vi "test.vi"() -> ()   [LabVIEW 2014]
uses:
  Array-Parameter/_support/Def-MassDataOper-Status.ctl
  Array-Parameter/_support/Operation-FGV-MassData.ctl
  Array-Parameter/JKISM++ Array Parameter Support.lvlib
panel:
  out "Waveform Graph":dbl[](graph)
  in  "Start":i32
  in  "read":bool
  out "Thermometer":cluster{dbl, dbl, dbl, dbl}(slide)={0.0, 6224.489795918367, 0.0, 0.0} scale=0.0..10000000.0
  in  "write":bool
  out "Active Read Oper":T1
  out "Active Write Oper":T1
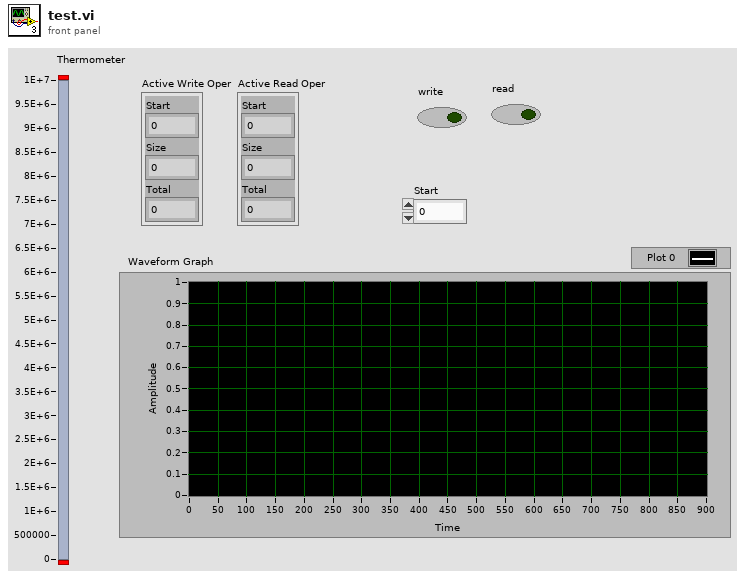
[diagram p1: front panel]
types:
  T1 = typedef "JKISM++ Array Parameter Support.lvlib/Def-MassDataOper-Status.ctl" = cluster{"Start":i32, "Size":i32, "Total":i32}
  T2 = typedef "JKISM++ Array Parameter Support.lvlib/Operation-FGV-MassData.ctl" = enum16{"Initialize", "Read", "Write", "Status", "Release"}
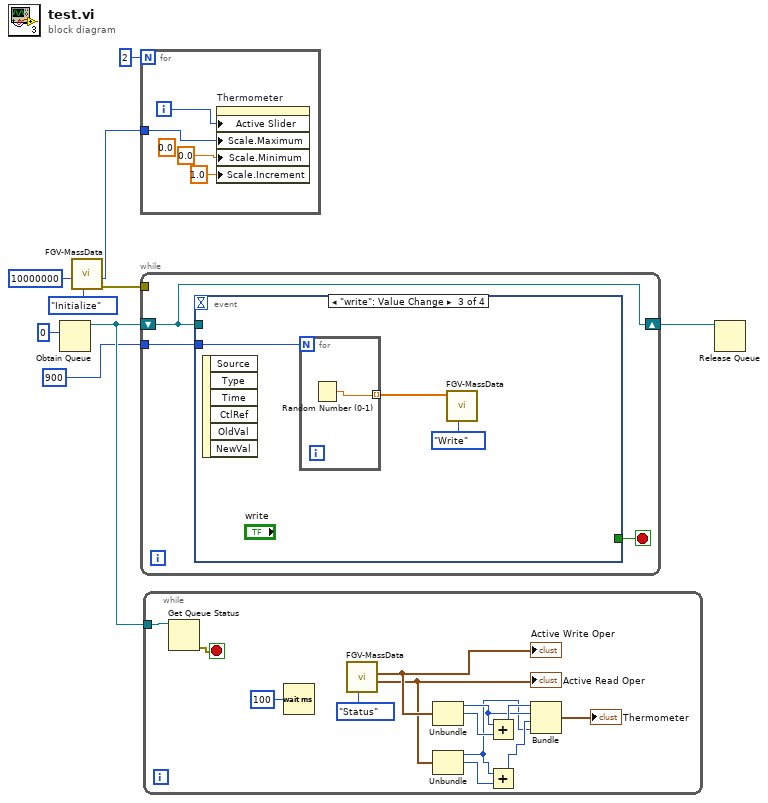
[diagram p0: block diagram]
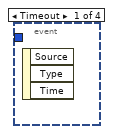
[diagram p2: hidden frame]
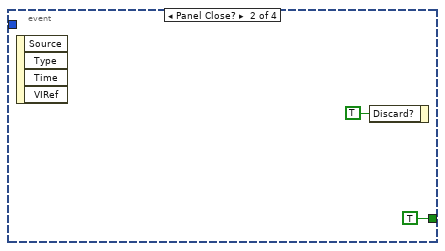
[diagram p3: hidden frame]
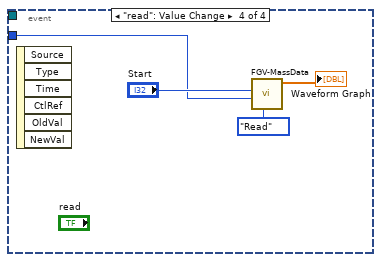
[diagram p4: hidden frame]
diagram:
  w2 = 10000000 ("size")
  n1 = Obtain Queue(element data type=0 ("size")) -> (queue out=w5:refnum<queue>)  [unwired: 4 in, 2 out]
  n2 = call "FGV-MassData.vi"("Operation"=Operation-FGV-MassData."Initialize", "size"=w2) -> ("Error out"=w7:errorcluster)  [unwired: 6 in, 3 out]
  n3 = for {
    N: 2 -> [_]
    tunnel: w2 -> [w10]
    i -> [w9]
    (unwired) 0.0 ("Scale.Range:Minimum")
    n4 = property on="Thermometer" class="Slide (strict)"("Active Slider"=w9, "Scale.Maximum"=w10, "Scale.Minimum"=0.0 ("Scale.Range:Minimum"), "Scale.Increment"=1.0 ("Scale.Range:Increment")) -> ()  [unwired: 2 in, 2 out]
  }
  n5 = while {
    tunnel: w7 -> [_]
    shift-right: [w14] -> w6
    shift-left: w5 -> [w14]
    tunnel: 900 -> [w13]
    stop <- w15 stop-if-true
    n6 = event shown="[2] \"write\": Value Change" {
      selector: _ -> [_ _ _ _]
      dyn-events: _ -> [_ _ _ _]
      timeout: _ -> [_ _ _ _]
      tunnel: [_ TRUE ("Discard?") _ _] -> w15
      tunnel: w14 -> [_ _ _ _]
      tunnel: w13 -> [_ _ w18 w23]
      event Timeout {
        n7 = event-data() -> ()  [unwired: 1 in, 3 out]
      }
      event Panel Close? {
        n8 = event-data() -> ()  [unwired: 1 in, 4 out]
        n9 = event-data("Discard?"=TRUE) -> ()  [unwired: 1 in, 1 out]
      }
      event "write": Value Change {
        n10 = event-data() -> ()  [unwired: 1 in, 6 out]
        n11 = for {
          N: w18 -> [_]
          tunnel: [w21] -> w19 mode=indexing
          n12 = Random Number (0-1)() -> (number: 0 to 1=w21:dbl)
        }
        n13 = call "FGV-MassData.vi"("Operation"=Operation-FGV-MassData."Write", "Data in"=w19) -> ()  [unwired: 6 in, 4 out]
      }
      event "read": Value Change {
        n14 = event-data() -> ()  [unwired: 1 in, 6 out]
        n15 = call "FGV-MassData.vi"("Operation"=Operation-FGV-MassData."Read", "size"=w23, "Start"="Start") -> ("Data out"=→"Waveform Graph":dbl[])  [unwired: 5 in, 3 out]
      }
    }
  }
  n16 = while {
    tunnel: w5 -> [w38]
    stop <- w37 stop-if-true
    n17 = Get Queue Status(queue=w38) -> (error out=w37:errorcluster)  [unwired: 2 in, 7 out]
    n18 = Wait (ms)(milliseconds to wait=u32 100) -> ()  [unwired: 1 out]
    n19 = call "FGV-MassData.vi"("Operation"=Operation-FGV-MassData."Status") -> ("Active Read Oper"=w29:T1, "Active Write Oper"=w34:T1)  [unwired: 7 in, 2 out]
    "Active Write Oper" <- w34
    "Active Read Oper" <- w29
    n20 = Unbundle(w34) -> ("Start"=w31:i32, "Size"=w33:i32)  [unwired: 1 out]
    n21 = Unbundle(w29) -> ("Start"=w27:i32, "Size"=w30:i32)  [unwired: 1 out]
    n22 = Add(x=w31, y=w33) -> (x+y=w32:i32)
    n23 = Add(x=w27, y=w30) -> (x+y=w28:i32)
    n24 = Bundle(w32, "Start"=w31, w28, "Start"=w27) -> (→"Thermometer":cluster{i32, "Start":i32, i32, "Start":i32})  [unwired: 1 in]
  }
  n25 = Release Queue(queue=w6) -> ()  [unwired: 2 in, 3 out]
